vi "Create_Filename.vi"(8 "error in (no error)":errorcluster, 11 "Test string input":string) -> (0 "error out":errorcluster, 3 "path for csv file":path)   [LabVIEW 2023]
uses:
  <vilib>/Utility/error.llb/whitespace.ctl
  <vilib>/Utility/error.llb/Trim Whitespace One-Sided.vi
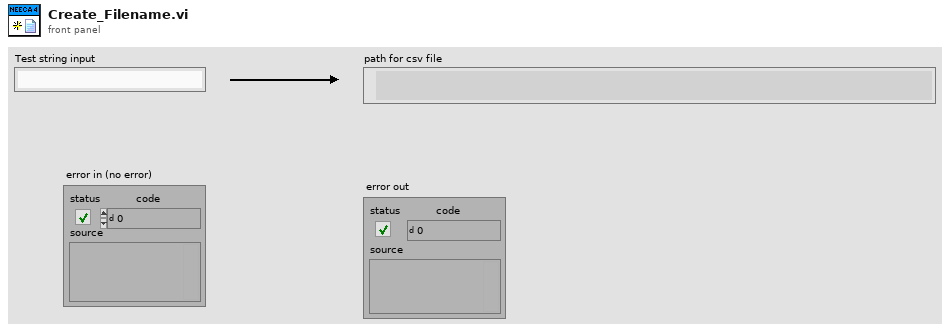
[diagram p1: front panel]
types:
  T1 = typedef "whitespace.ctl" = u16
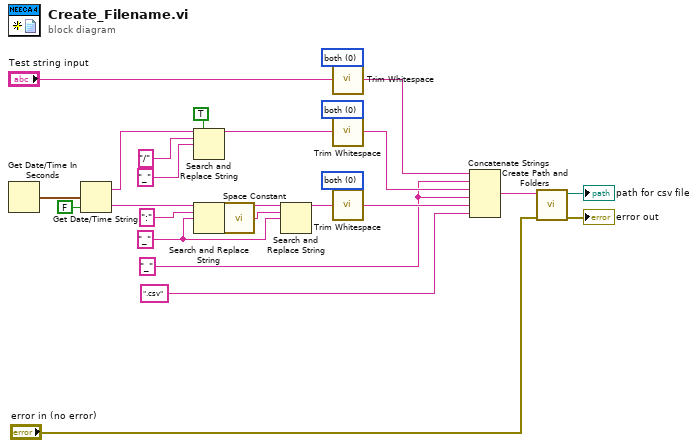
[diagram p0: block diagram]
diagram:
  w9 = T1 0 items=["both", "start of string", "end of string"] ("location (both)")
  w12 = T1 0 items=["both", "start of string", "end of string"] ("location (both)")
  w14 = T1 0 items=["both", "start of string", "end of string"] ("location (both)")
  w15 = "_" ("replace string (\"\")")
  w6 = "_"
  n1 = Get Date/Time In Seconds() -> (seconds since 1Jan1904=w24:timestamp)
  n2 = Get Date/Time String(seconds (now)=w24, want seconds? (F)=FALSE) -> (date string=w21:string, time string=w26:string)  [unwired: 1 in]
  n3 = Search and Replace String(replace all?=TRUE ("replace all? (F)"), input string=w21, search string="/", replace string="_" ("replace string (\"\")")) -> (result string=w11:string)  [unwired: 4 in, 3 out]
  n4 = Search and Replace String(input string=w26, search string=":", replace string=w15) -> (result string=w17:string)  [unwired: 5 in, 3 out]
  n5 = call <vilib>:"Space Constant.vi"() -> ("String"=w16:string)
  n6 = Search and Replace String(input string=w17, search string=w16, replace string=w15) -> (result string=w8:string)  [unwired: 5 in, 3 out]
  n7 = call <vilib>:"Trim Whitespace.vi"("string"="Test string input", "location (both)"=w14) -> ("trimmed string"=w13:string)
  n8 = call <vilib>:"Trim Whitespace.vi"("string"=w11, "location (both)"=w12) -> ("trimmed string"=w10:string)
  n9 = call <vilib>:"Trim Whitespace.vi"("string"=w8, "location (both)"=w9) -> ("trimmed string"=w7:string)
  n10 = Concatenate Strings(w13, w6, w10, w6, w7, ".csv" ("string")) -> (w4:string)
  n11 = call "Create Path and Folders.vi"("error in (no error)"="error in (no error)", "String Path"=w4) -> ("error out"=→"error out":errorcluster, "path for csv file"=→"path for csv file":path)  [unwired: 8 in]
